vi "SendCommand.vi"(4 "Wait Before Read (Ms)":u32=50, 6 "Timeout (Sec)":u32=500, 8 "error in":errorcluster, 10 "Command":string, 11 "Comport":refnum<visa-resource-name>="COM8") -> (0 "error out":errorcluster, 1 "Last Reply Entry":string, 2 "Reply":string, 3 "Comport Out":refnum<visa-resource-name>)   [LabVIEW 2020, in "MicroPythonClient.lvlib"]
doc: "Sends a command to a micropython target. The VI adds \"\\r\" to a non control message.\nTimeout (Sec) indicates that if, in a new receive cycle, we haven't received from the device and this timeout has been reached since we started listening, we will assume that the device is done talking.\nWait Before Read (Ms) indicates how long we should wait before checking the receive buffer at the beginning of a receive cycle."
uses:
  MicroPythonClient.lvlib
  <vilib>/regexp/Match Regular Expression.xnode
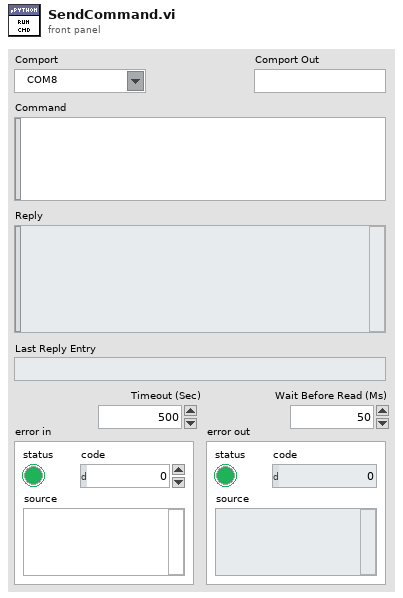
[diagram p1: front panel]
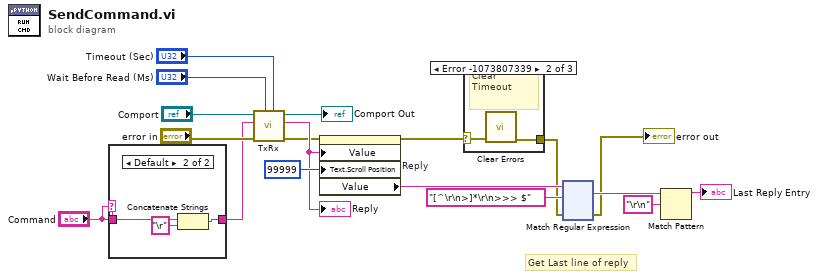
[diagram p0: block diagram]
diagram:
  # "Get Last line of reply"
  n1 = case shown="Default" "Command" {
    selector: "Command" -> [_ w20]
    tunnel: "Command" -> [w19 _]
    tunnel: [w19 w21] -> w5
    frame "\u0001", "\u0002", "\u0003", "\u0004", "\u0005" {
      # "control cmds\nctrl +a\n...\nctrl + e"
    }
    frame Default {
      n2 = Concatenate Strings(w20, "\r" ("string")) -> (w21:string)
    }
  }
  n3 = call "TxRx.vi"("Timeout (Ms)"="Timeout (Sec)", "Wait Before Read (Ms)"="Wait Before Read (Ms)", "error in"="error in", "Tx Message"=w5, "VISA Resource Name In"="Comport") -> ("error out"=w2:errorcluster, "Rx Message"=w13:string, "VISA Resource Name Out"=→"Comport Out":refnum<visa-resource-name>)  [unwired: 4 in]
  "Reply" <- w13
  n4 = property on="Reply" class="Str"(error in=w2, "Value"=w13, "Text.Scroll Position"=u32 99999 ("byte count")) -> (error out=w1:errorcluster, "Value"=w7:string)  [unwired: 1 in, 1 out]
  n5 = case shown="Error -1073807339" w1 {
    selector: w1 -> [w23 w25 w26]
    tunnel: [w23 w24 w26] -> w4
    frame No Error {
    }
    frame Error {
      # "Clear Timeout"
      n6 = call <vilib>:"Clear Errors.vi"("error in (no error)"=w25) -> ("error out"=w24:errorcluster)  [unwired: 5 in, 1 out]
    }
    frame Default {
    }
  }
  n7 = xnode "Match Regular Expression"("input string"=w7, "regular expression"="[^\r\n>]*\r\n>>> $", "error in"=w4) -> ("whole match"=w17:string, "error out"=→"error out":errorcluster)  [unwired: 3 in, 3 out]
  n8 = Match Pattern(string=w17, regular expression="\r\n") -> (before substring=→"Last Reply Entry":string)  [unwired: 1 in, 3 out]
